vi "Read Gui_TestCtrl.vi"(8 "error in (no error)":errorcluster, 11 "GUI_Handler_Seq in":refnum<class "GUI_Handler_Seq.lvclass">) -> (0 "error out":errorcluster, 2 "Gui_TestCtrl":T1, 3 "GUI_Handler_Seq out":refnum<class "GUI_Handler_Seq.lvclass">)   [LabVIEW 2017, in "GUI_Handler_Seq.lvclass"]
uses:
  GUI_Handler_Seq.lvclass
  GUI_Handler_Seq.lvclass/GUI_Handler_Seq.ctl
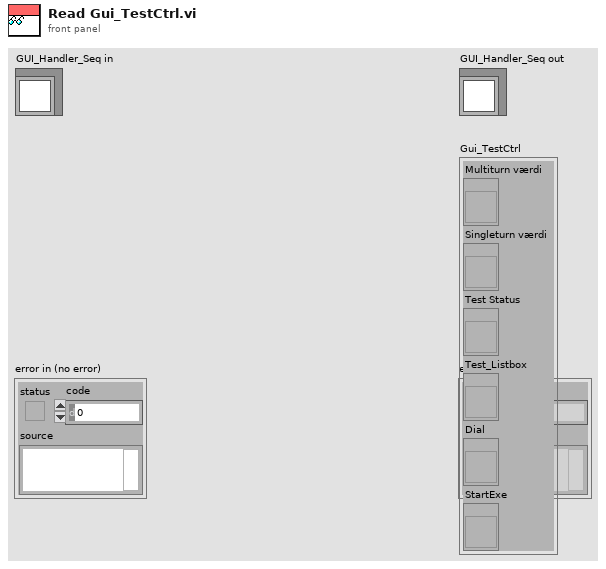
[diagram p1: front panel]
types:
  T1 = cluster{"Multiturn værdi":refnum<vi>, "Singleturn værdi":refnum<vi>, "Test Status":refnum<vi>, "Test_Listbox":refnum<vi>, "Dial":refnum<vi>, "StartExe":refnum<vi>}
  T2 = cluster{"Multiturn værdi":refnum<vi>, "Singleturn værdi":refnum<vi>, "Status":refnum<vi>, "Seq_Listbox":refnum<vi>, "Dial":refnum<vi>, "StartExe":refnum<vi>}
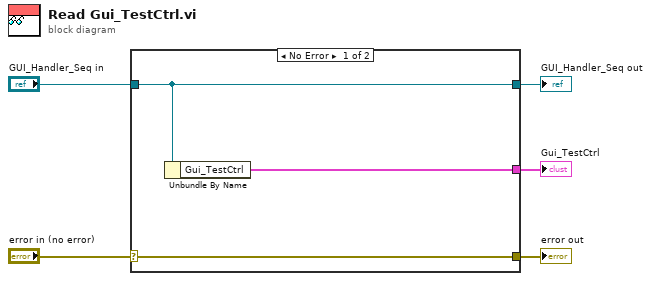
[diagram p0: block diagram]
diagram:
  n1 = case shown="No Error" "error in (no error)" {
    selector: "error in (no error)" -> [w8 w9]
    tunnel: [w8 w9] -> w4
    tunnel: [w7 w10] -> w2
    tunnel: "GUI_Handler_Seq in" -> [w7 w10]
    tunnel: [w6 _] -> w1
    frame No Error {
      n2 = Unbundle By Name(w7) -> ("Gui_TestCtrl"=w6:T2)
    }
    frame Error {
    }
  }
  "error out" <- w4
  "GUI_Handler_Seq out" <- w2
  "Gui_TestCtrl" <- w1
